vi "Eat.vi"(8 "error in (no error)":errorcluster, 10 "String":string, 11 "Tiger in":refnum<class "Tiger.lvclass">) -> (0 "error out":errorcluster, 2 "String 2":string, 3 "Tiger out":refnum<class "Tiger.lvclass">)   [LabVIEW 2018, in "Tiger.lvclass"]
uses:
  Tiger.lvclass
  animal/Animal.lvclass
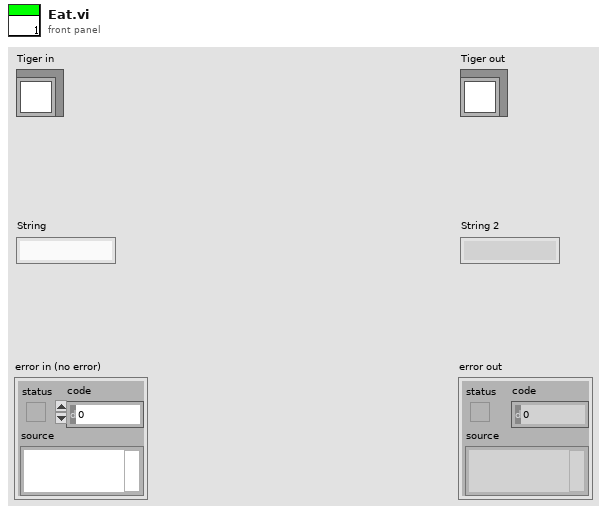
[diagram p1: front panel]
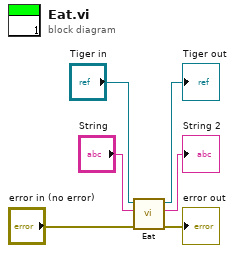
[diagram p0: block diagram]
diagram:
  n1 = call-parent "Eat.vi"("error in (no error)"="error in (no error)", "String"="String", "Animal in"="Tiger in") -> ("error out"=→"error out":errorcluster, "String 2"=→"String 2":string, "Animal out"=→"Tiger out":refnum<class "Tiger.lvclass">)  [unwired: 6 in]
